vi "read_data.vi"(8 "error in (no error)":errorcluster, 11 "Lars in":refnum<class "Lars.lvclass">) -> (0 "error out":errorcluster, 2 "data":T1, 3 "Lars out":refnum<class "Lars.lvclass">)   [LabVIEW 2020, in "Lars.lvclass"]
uses:
  Lars.lvclass
  Controls/lars_data.ctl
  Lars.lvclass/Lars.ctl
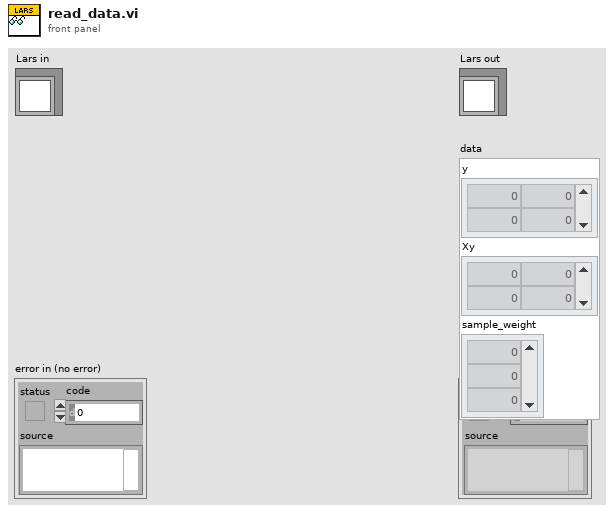
[diagram p1: front panel]
types:
  T1 = typedef "lars_data.ctl" = cluster{"y":dbl[][], "Xy":dbl[][], "sample_weight":dbl[]}
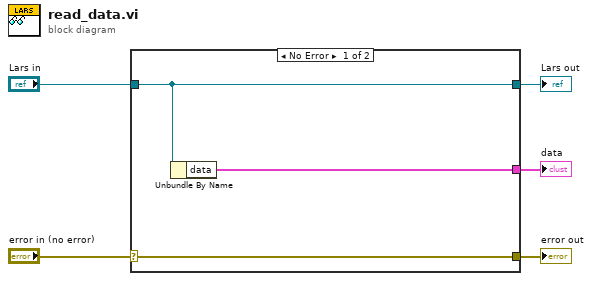
[diagram p0: block diagram]
diagram:
  n1 = case shown="No Error" "error in (no error)" {
    selector: "error in (no error)" -> [w8 w9]
    tunnel: [w8 w9] -> w4
    tunnel: [w7 w10] -> w2
    tunnel: "Lars in" -> [w7 w10]
    tunnel: [w6 _] -> w1
    frame No Error {
      n2 = Unbundle By Name(w7) -> ("data"=w6:T1)
    }
    frame Error {
    }
  }
  "error out" <- w4
  "Lars out" <- w2
  "data" <- w1
